vi "Get Version Info.vi"(8 "error in (no error)":errorcluster, 9 "ui32BufferLen":u32, 10 "szVersionInfo":string, 11 "arr":u32(ring)=65535 items=["AT_SDKVersion"=1073741824, "AT_DeviceDriverVersion"=1073741825]) -> (0 "error out":errorcluster, 2 "szVersionInfo out":string, 3 "function return":u32)   [LabVIEW 2014, in "atmcd32d.lvlib"]
doc: "unsigned int WINAPI GetVersionInfo(AT_VersionInfoId arr, char * szVersionInfo, at_u32 ui32BufferLen);"
uses:
  atmcd32d.lvlib
  atmcd32d.dll
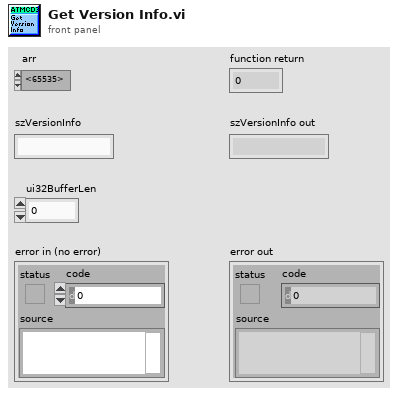
[diagram p1: front panel]
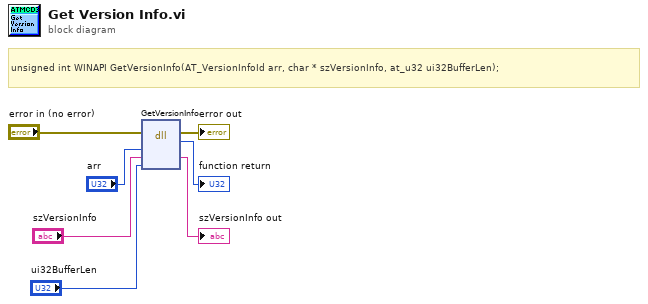
[diagram p0: block diagram]
diagram:
  # "unsigned int WINAPI GetVersionInfo(AT_VersionInfoId arr, char * szVersionInfo, at_u32 ui32BufferLen);"
  n1 = dll-call lib="C:/Users/Bakir/Documents/Lambda2-Testing/lib/Andorlib/atmcd32d.*" fn="GetVersionInfo"(error in="error in (no error)", "arr"="arr", "szVersionInfo"="szVersionInfo", "ui32BufferLen"="ui32BufferLen") -> (error out=→"error out":errorcluster, →"function return":u32, "szVersionInfo"=→"szVersionInfo out":string)  [unwired: 4 in, 1 out]
